vi "Main.vi"() -> ()   [LabVIEW 2018]
doc: "This Continuous Measurement sample project is based on the Queued Message Handler template.\n\nThe Event Handling Loop generates messages based on user interface actions.\n\nThe Message Handling Loop processes messages generated by the Event Handling Loop, or by other messages. There are also Acquisition and Logging message handling loop subVIs, and a chart updating loop."
uses:
  Controls/Acquired Data.ctl
  Settings/Settings.ctl
  Acquisition/Hardware Configuration.ctl
  Acquisition/Signal Type.ctl
  Logging/Logging Configuration.ctl
  Controls/UI State.ctl
  Support/Message Queue/Enqueue Message (Single).vi
  Support/Message Queue/Enqueue Message (Array).vi
  <vilib>/Utility/error.llb/Error Cluster From Error Code.vi
  <vilib>/ErrorRing/Error Ring.xnode
  Acquisition/Acquisition.lvlib
  Logging/Logging.lvlib
  Settings/Settings.lvlib
  support/User Event - Stop/User Event - Stop.lvlib
  support/Message Queue/Message Queue.lvlib
  Settings/Settings Dialog.vi
  Data Display/Data Display.lvlib
panel:
  in  "Data":T1
  out "User Event - Stop":refnum<user-event>
  out "Data":T1(graph)
  in  "Settings":bool
  in  "Start":bool
  in  "Stop":bool
  out "Status":string
  in  "Exit":bool
  # "Continuous Measurement Data Logger"
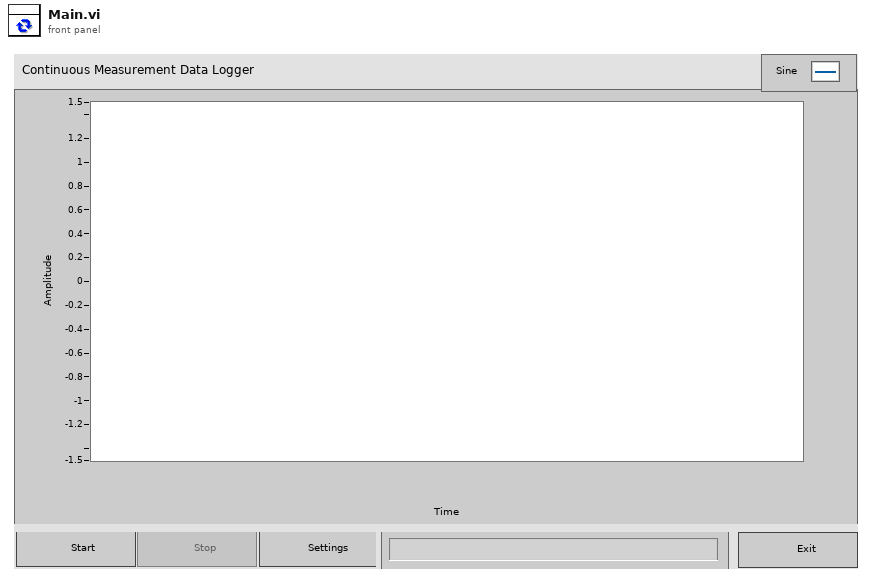
[diagram p1: front panel]
types:
  T1 = typedef "Acquired Data.ctl" = waveform(dbl)[]
  T2 = typedef "UI State.ctl" = enum16{"Idle", "Acquiring and Logging", "Waiting for Exit", "Waiting for Exit (Acq Stopped)", "Waiting for Exit (Log Stopped)", "Waiting for Stop", "Waiting for Stop (Acq Stopped)", "Waiting for Stop (Log Stopped)"}
  T3 = typedef "Settings.lvlib/Settings.ctl" = cluster{"Hardware Configuration":T4, "Logging Configuration":T6, "UI Refs":cluster{"Start Ref":refnum<vi>, "Settings Ref":refnum<vi>, "Stop Ref":refnum<vi>, "Exit Ref":refnum<vi>, "Status Ref":refnum<vi>, "Data Ref":refnum<vi>}}
  T4 = typedef "Acquisition.lvlib/Hardware Configuration.ctl" = cluster{"HW Refnum <Replace Me>":string, "Signal Type <Replace Me>":T5}
  T5 = typedef "Acquisition.lvlib/Signal Type.ctl" = enum16{"Sine Wave", "Square with Noise"}
  T6 = typedef "Logging.lvlib/Logging Configuration.ctl" = cluster{"Log File Base Path":path, "TDMS File Reference":refnum<k34>}
  T7 = typedef "Message Queue.lvlib/All Message Queues.ctl" = cluster{"Message Queues":cluster{"UI":refnum<queue>, "Acquisition":refnum<queue>, "Logging":refnum<queue>}, "Data Queues & Notifier":cluster{"Data Queue":T8, "Data Notifer":T9}}
  T8 = typedef "Data Queue.ctl" = refnum<queue>
  T9 = typedef "Data Notifier.ctl" = refnum<notifier>
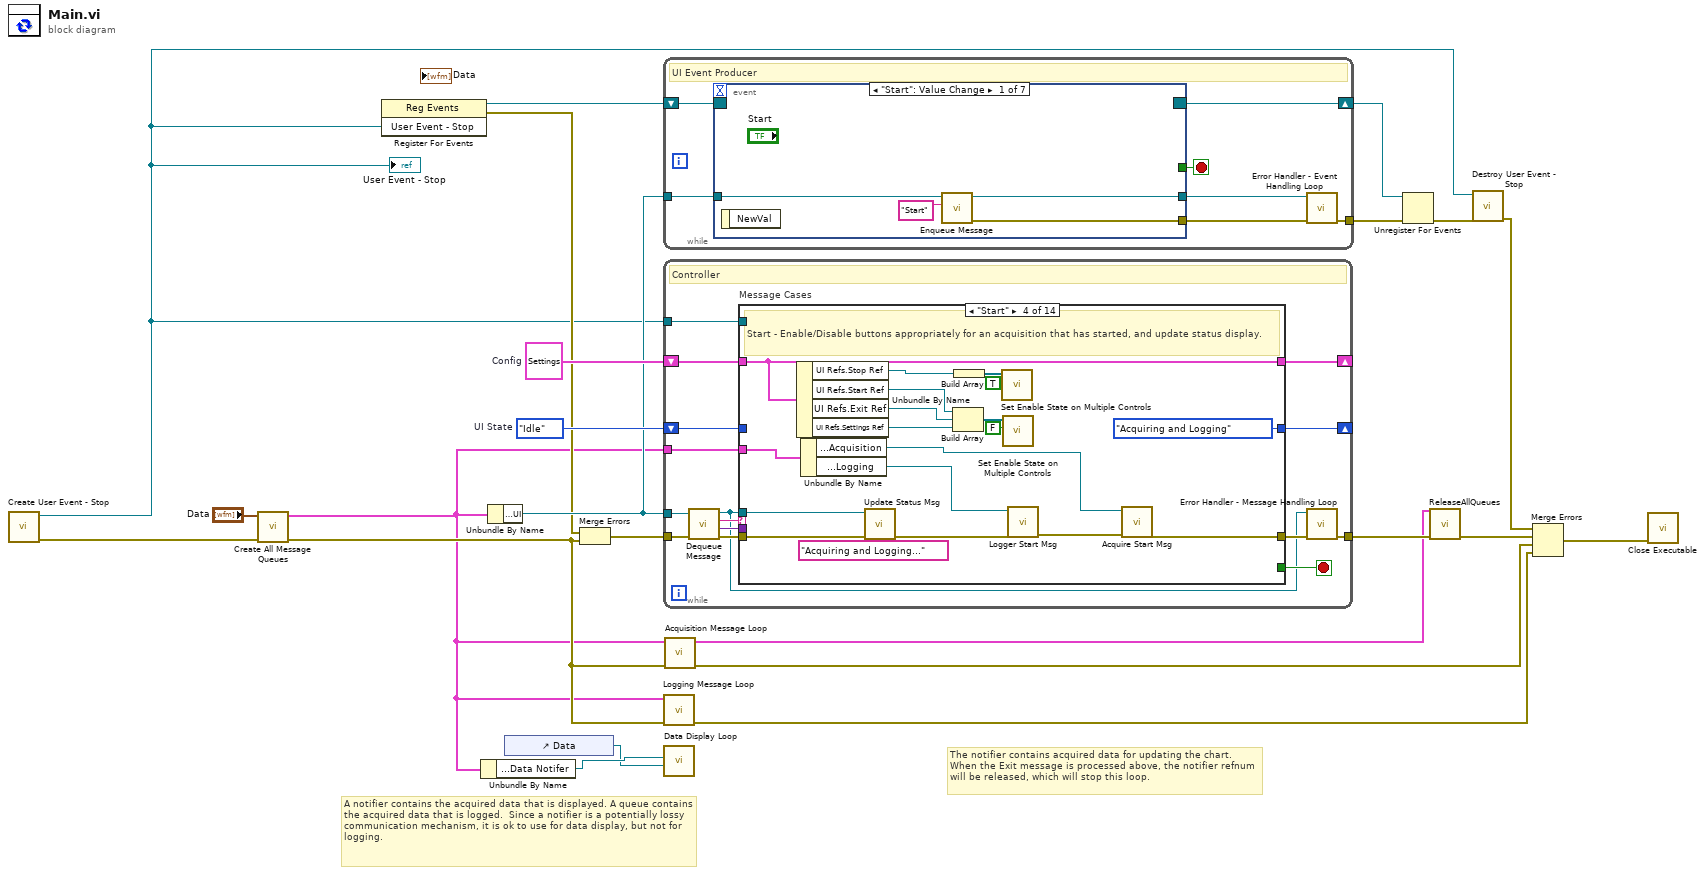
[diagram p0: block diagram]
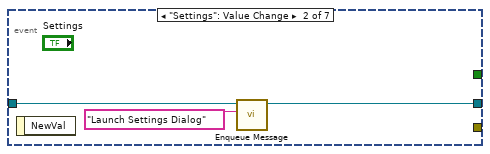
[diagram p2: hidden frame]
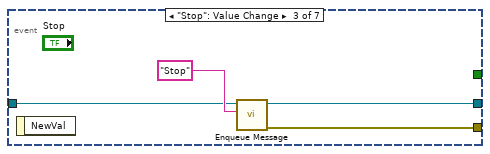
[diagram p3: hidden frame]
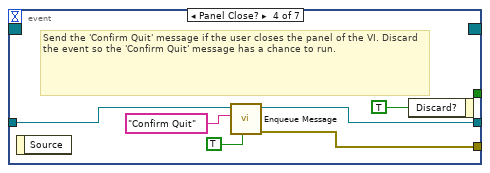
[diagram p4: hidden frame]
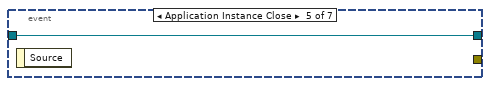
[diagram p5: hidden frame]
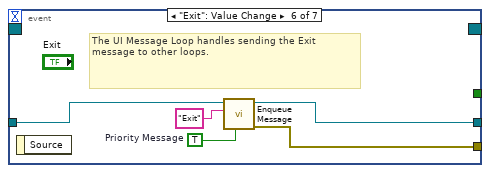
[diagram p6: hidden frame]
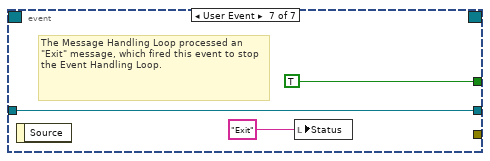
[diagram p7: hidden frame]
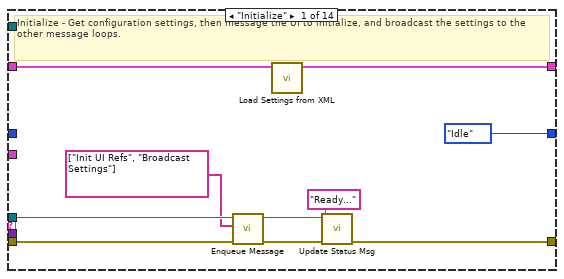
[diagram p8: hidden frame]
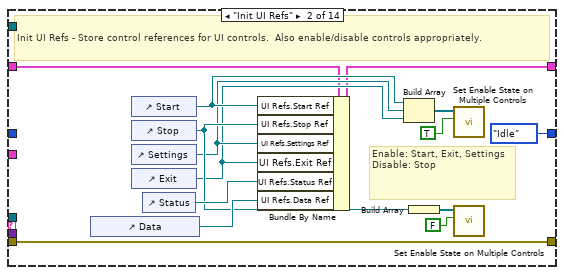
[diagram p9: hidden frame]
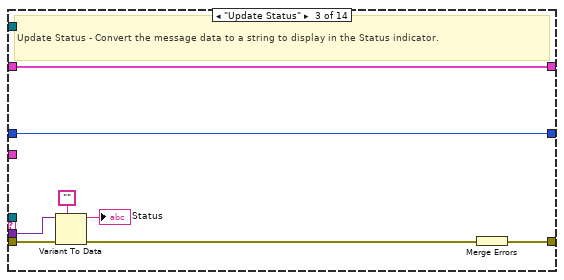
[diagram p10: hidden frame]
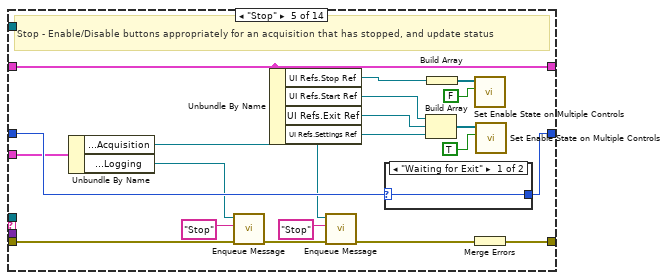
[diagram p11: hidden frame]
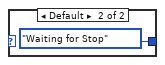
[diagram p12: hidden frame]
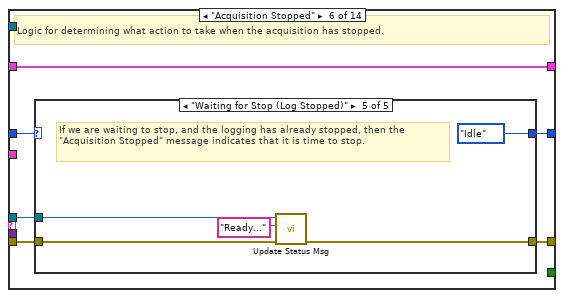
[diagram p13: hidden frame]
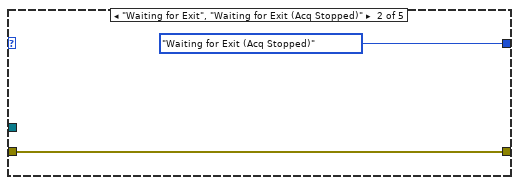
[diagram p15: hidden frame]
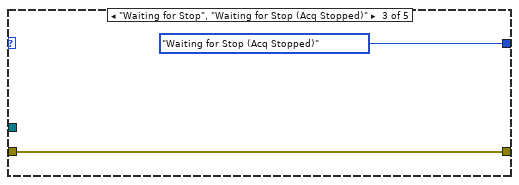
[diagram p16: hidden frame]
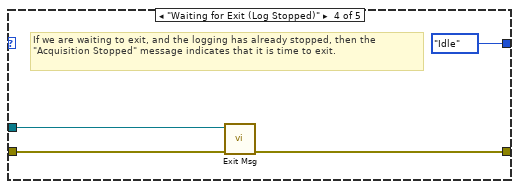
[diagram p17: hidden frame]
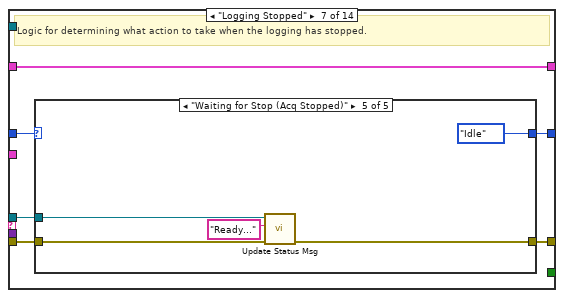
[diagram p18: hidden frame]
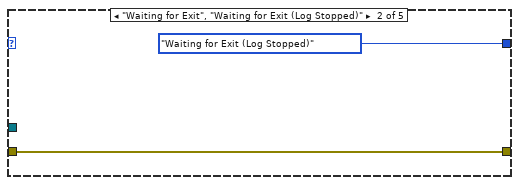
[diagram p20: hidden frame]
diagram:
  w14 = UI_State."Idle"  # UI State
  w16 = T3 {"Hardware Configuration"={"HW Refnum <Replace Me>"="", "Signal Type <Replace Me>"=enum."Sine Wave"}, "Logging Configuration"={"Log File Base Path"=path "", "TDMS File Reference"=refnum}, "UI Refs"={"Start Ref"=refnum, "Settings Ref"=refnum, "Stop Ref"=refnum, "Exit Ref"=refnum, "Status Ref"=refnum, "Data Ref"=refnum}}  # Config
  # "A notifier contains the acquired data that is displayed. A queue contains the acquired data that is logged.  Since a notifier is a potentially lossy communication mechanism, it is ok to use for data display, but not for logging."
  # "The notifier contains acquired data for updating the chart. When the Exit message is processed above, the notifier refnum will be released, which will stop this loop."
  n1 = call "Create User Event - Stop.vi"() -> ("error out"=w19:errorcluster, "User Event - Stop"=w8:refnum<user-event>)  [unwired: 10 in]
  "User Event - Stop" <- w8
  n2 = call "Create All Message Queues.vi"("error in (no error)"=w19, "Data"="Data") -> ("error out"=w17:errorcluster, "Message Queues out"=w5:T7)  [unwired: 8 in]
  n3 = register-events(w8) -> (reference out=w11:refnum<event-registration>, error out=w9:errorcluster)  [unwired: 2 in]
  n4 = Unbundle By Name(w5) -> ("Data Queues & Notifier.Data Notifer"=w7:T9)
  n5 = Unbundle By Name(w5) -> ("Message Queues.UI"=w13:refnum<queue>)
  n6 = control-ref of="Data"() -> (w1:refnum<vi>)
  n7 = Merge Errors(w9, w17) -> (w10:errorcluster)
  n8 = while {
    tunnel: w13 -> [w28]
    tunnel: [w25] -> w21
    shift-right: [w27] -> w15
    shift-left: w11 -> [w29]
    stop <- w26 stop-if-true
    # "UI Event Producer"
    n9 = event shown="[0] \"Start\": Value Change" {
      selector: w29 -> [_ _ _ _ _ _ _]
      dyn-events: [_ _ _ _ _ _ _] -> w27
      timeout: _ -> [_ _ _ _ _ _ _]
      tunnel: [_ _ _ _ _ _ TRUE ("Discard?")] -> w26
      tunnel: w28 -> [w33 w35 w39 w44 w47 w49 w53]
      tunnel: [w31 _ w38 w42 _ w52 _] -> w24
      tunnel: [w30 w34 w37 w43 w47 w48 w53] -> w23
      event "Start": Value Change {
        n10 = event-data() -> ()  [unwired: 1 in, 1 out]
        n11 = call-poly "Enqueue Message.vi"("Message"="Start", "Message Queue"=w33) -> ("error out"=w31:errorcluster, "dup Message Queue"=w30:refnum<queue>)  [unwired: 8 in]
      }
      event "Settings": Value Change {
        n12 = event-data() -> ()  [unwired: 1 in, 1 out]
        n13 = call-poly "Enqueue Message.vi"("Message"="Launch Settings Dialog", "Message Queue"=w35) -> ("dup Message Queue"=w34:refnum<queue>)  [unwired: 8 in, 1 out]
      }
      event "Stop": Value Change {
        n14 = event-data() -> ()  [unwired: 1 in, 1 out]
        n15 = call-poly "Enqueue Message.vi"("Message"="Stop", "Message Queue"=w39) -> ("error out"=w38:errorcluster, "dup Message Queue"=w37:refnum<queue>)  [unwired: 8 in]
      }
      event Panel Close? {
        # "Send the 'Confirm Quit' message if the user closes the panel of the VI. Discard the event so the 'Confirm Quit' message has a chance to run."
        n16 = event-data() -> ()  [unwired: 1 in, 1 out]
        n17 = call-poly "Enqueue Message.vi"("Priority Message? (F)"=TRUE, "Message"="Confirm Quit", "Message Queue"=w44) -> ("error out"=w42:errorcluster, "dup Message Queue"=w43:refnum<queue>)  [unwired: 7 in]
        n18 = event-data("Discard?"=TRUE) -> ()  [unwired: 1 in, 1 out]
      }
      event Application Instance Close {
        n19 = event-data() -> ()  [unwired: 1 in, 1 out]
      }
      event "Exit": Value Change {
        w50 = TRUE  # Priority Message
        # "The UI Message Loop handles sending the Exit message to other loops."
        n20 = event-data() -> ()  [unwired: 1 in, 1 out]
        n21 = call-poly "Enqueue Message.vi"("Priority Message? (F)"=w50, "Message"="Exit", "Message Queue"=w49) -> ("error out"=w52:errorcluster, "dup Message Queue"=w48:refnum<queue>)  [unwired: 7 in]
      }
      event User Event {
        # "The Message Handling Loop processed an \"Exit\" message, which fired this event to stop the Event Handling Loop."
        n22 = event-data() -> ()  [unwired: 1 in, 1 out]
        n23 = local write "Status"("Exit" ("Exit String")) -> ()
      }
    }
    n24 = call "Error Handler - Event Handling Loop.vi"("error in (no error)"=w24, "Message Queue"=w23) -> ("dup error in"=w25:errorcluster)  [unwired: 8 in, 1 out]
  }
  n25 = while {
    tunnel: w13 -> [w64]
    tunnel: w8 -> [w69]
    shift-right: [w63] -> _
    shift-left: w16 -> [w62]
    shift-right: [w57] -> _
    shift-left: w14 -> [w58]
    tunnel: w10 -> [w68]
    tunnel: [w61] -> w22
    tunnel: w5 -> [w56]
    stop <- w70 stop-if-true
    # "Controller"
    n26 = call "Dequeue Message.vi"("error in (no error)"=w68, "Message Queue"=w64) -> ("error out"=w67:errorcluster, "Message Data"=w65:variant, "Message"=w66:string, "dup Message Queue"=w59:refnum<queue>)  [unwired: 6 in]
    n27 = case "Message Cases" shown="\"Start\"" w66 {
      selector: w66 -> [_ _ _ _ _ _ _ _ _ _ _ _ _ w266]
      tunnel: w59 -> [w78 _ _ w106 _ w146 w167 _ w202 _ w221 _ _ _]
      tunnel: w67 -> [w77 w94 w101 w105 w140 w147 w168 w191 w204 w210 w220 w251 w264 _]
      tunnel: [w71 w94 w102 w112 w141 w144 w165 w197 w198 w213 w219 w258 w263 w265] -> w60
      tunnel: [_ _ _ _ _ _ _ _ _ _ _ TRUE _ _] -> w70
      tunnel: w65 -> [_ _ w100 _ _ _ _ _ _ w214 _ w249 _ _]
      tunnel: w69 -> [_ _ _ _ _ _ _ _ _ _ _ w259 _ _]
      tunnel: [w79 w81 w96 w110 w125 w149 w170 w195 w201 w217 w223 w257 w262 w268] -> w63
      tunnel: w62 -> [w80 w82 w96 w110 w125 w149 w170 w195 w205 w217 w223 w257 w262 w268]
      tunnel: w58 -> [_ _ w95 _ w126 w148 w169 w189 w199 w212 w222 _ w261 w267]
      tunnel: [UI_State."Idle" ("UI State") UI_State."Idle" ("UI State") w95 UI_State."Acquiring and Logging" ("UI State") w127 w145 w166 w189 w199 w212 w218 UI_State."Idle" ("UI State") w261 w267] -> w57
      tunnel: w56 -> [_ _ _ w109 w124 _ _ w188 _ _ _ w247 _ _]
      frame "Initialize" {
        # "Initialize - Get configuration settings, then message the UI to initialize, and broadcast the settings to the other message loops."
        n28 = call-poly "Enqueue Message.vi"("error in (no error)"=w77, "Message Array"=string[] ["Init UI Refs", "Broadcast Settings"], "Message Queue"=w78) -> ("error out"=w72:errorcluster, "dup Message Queue"=w74:refnum<queue>)  [unwired: 7 in]
        n29 = call "Load Settings from XML.vi"("Settings in"=w80) -> ("Settings out"=w79:T3)  [unwired: 9 in, 1 out]
        n30 = call "Update Status Msg.vi"("error in (no error)"=w72, "Ready..."="Ready...", "Queue in"=w74) -> ("error out"=w71:errorcluster)  [unwired: 8 in]
      }
      frame "Init UI Refs" {
        # "Enable: Start, Exit, Settings\nDisable: Stop"
        # "Init UI Refs - Store control references for UI controls.  Also enable/disable controls appropriately."
        n31 = control-ref of="Data"() -> (w92:refnum<vi>)
        n32 = control-ref of="Start"() -> (w86:refnum<vi>)
        n33 = control-ref of="Stop"() -> (w87:refnum<vi>)
        n34 = control-ref of="Settings"() -> (w85:refnum<vi>)
        n35 = control-ref of="Exit"() -> (w84:refnum<vi>)
        n36 = control-ref of="Status"() -> (w93:refnum<vi>)
        n37 = Bundle By Name(cluster=w82, "UI Refs.Start Ref"=w86, "UI Refs.Stop Ref"=w87, "UI Refs.Settings Ref"=w85, "UI Refs.Exit Ref"=w84, "UI Refs.Status Ref"=w93, "UI Refs.Data Ref"=w92) -> (w81:T3)
        n38 = Build Array(w86, w85, w84) -> (w90:refnum<vi>[])
        n39 = Build Array(w87) -> (w89:refnum<vi>[])
        n40 = call "Set Enable State on Multiple Controls.vi"("Enable?"=TRUE, "Controls"=w90) -> ()  [unwired: 10 in]
        n41 = call "Set Enable State on Multiple Controls.vi"("Enable?"=FALSE, "Controls"=w89) -> ()  [unwired: 10 in]
      }
      frame "Update Status" {
        # "Update Status - Convert the message data to a string to display in the Status indicator."
        n42 = Variant To Data(error in=w101, type="", Variant=w100) -> (data=→"Status":string, error out=w98:errorcluster)
        n43 = Merge Errors(w98) -> (w102:errorcluster)
      }
      frame "Start" {
        # "Start - Enable/Disable buttons appropriately for an acquisition that has started, and update status display."
        n44 = Unbundle By Name(w110) -> ("UI Refs.Stop Ref"=w117:refnum<vi>, "UI Refs.Start Ref"=w116:refnum<vi>, "UI Refs.Exit Ref"=w115:refnum<vi>, "UI Refs.Settings Ref"=w114:refnum<vi>)
        n45 = Unbundle By Name(w109) -> ("Message Queues.Acquisition"=w108:refnum<queue>, "Message Queues.Logging"=w107:refnum<queue>)
        n46 = call "Update Status Msg.vi"("error in (no error)"=w105, "Ready..."="Acquiring and Logging..." ("Acquiring and Logging..."), "Queue in"=w106) -> ("error out"=w104:errorcluster)  [unwired: 8 in]
        n47 = Build Array(w116, w115, w114) -> (w120:refnum<vi>[])
        n48 = Build Array(w117) -> (w119:refnum<vi>[])
        n49 = call "Set Enable State on Multiple Controls.vi"("Enable?"=TRUE, "Controls"=w119) -> ()  [unwired: 10 in]
        n50 = call "Set Enable State on Multiple Controls.vi"("Enable?"=FALSE, "Controls"=w120) -> ()  [unwired: 10 in]
        n51 = call "Logger Start Msg.vi"("error in (no error)"=w104, "Queue in"=w107) -> ("error out"=w113:errorcluster)  [unwired: 9 in]
        n52 = call "Acquire Start Msg.vi"("error in (no error)"=w113, "Queue in"=w108) -> ("error out"=w112:errorcluster)  [unwired: 9 in]
      }
      frame "Stop" {
        # "Stop - Enable/Disable buttons appropriately for an acquisition that has stopped, and update status"
        n53 = Unbundle By Name(w124) -> ("Message Queues.Acquisition"=w123:refnum<queue>, "Message Queues.Logging"=w122:refnum<queue>)
        n54 = call-poly "Enqueue Message.vi"("error in (no error)"=w140, "Message"="Stop", "Message Queue"=w122) -> ("error out"=w130:errorcluster)  [unwired: 7 in, 1 out]
        n55 = Unbundle By Name(w125) -> ("UI Refs.Stop Ref"=w135:refnum<vi>, "UI Refs.Start Ref"=w134:refnum<vi>, "UI Refs.Exit Ref"=w133:refnum<vi>, "UI Refs.Settings Ref"=w132:refnum<vi>)
        n56 = call-poly "Enqueue Message.vi"("error in (no error)"=w130, "Message"="Stop", "Message Queue"=w123) -> ("error out"=w129:errorcluster)  [unwired: 7 in, 1 out]
        n57 = case shown="\"Waiting for Exit\"" w126 {
          selector: w126 -> [w142 _]
          tunnel: [w142 UI_State."Waiting for Stop" ("UI State")] -> w127
          frame "Waiting for Exit" {
          }
          frame Default {
          }
        }
        n58 = Build Array(w134, w133, w132) -> (w138:refnum<vi>[])
        n59 = Build Array(w135) -> (w137:refnum<vi>[])
        n60 = call "Set Enable State on Multiple Controls.vi"("Enable?"=FALSE, "Controls"=w137) -> ()  [unwired: 10 in]
        n61 = Merge Errors(w129) -> (w141:errorcluster)
        n62 = call "Set Enable State on Multiple Controls.vi"("Enable?"=TRUE, "Controls"=w138) -> ()  [unwired: 10 in]
      }
      frame "Acquisition Stopped" {
        # "Logic for determining what action to take when the acquisition has stopped."
        n63 = case shown="\"Waiting for Stop (Log Stopped)\"" w148 {
          selector: w148 -> [w151 _ _ _ _]
          tunnel: w147 -> [w150 w153 w155 w158 w162]
          tunnel: w146 -> [_ _ _ w157 w163]
          tunnel: [w151 UI_State."Waiting for Exit (Acq Stopped)" ("UI State") UI_State."Waiting for Stop (Acq Stopped)" ("UI State") UI_State."Idle" ("UI State") UI_State."Idle" ("UI State")] -> w145
          tunnel: [w150 w153 w155 w156 w161] -> w144
          frame Default {
          }
          frame "Waiting for Exit", "Waiting for Exit (Acq Stopped)" {
          }
          frame "Waiting for Stop", "Waiting for Stop (Acq Stopped)" {
          }
          frame "Waiting for Exit (Log Stopped)" {
            # "If we are waiting to exit, and the logging has already stopped, then the \"Acquisition Stopped\" message indicates that it is time to exit."
            n64 = call "Exit Msg.vi"("error in (no error)"=w158, "Queue in"=w157) -> ("error out"=w156:errorcluster)  [unwired: 9 in]
          }
          frame "Waiting for Stop (Log Stopped)" {
            # "If we are waiting to stop, and the logging has already stopped, then the \"Acquisition Stopped\" message indicates that it is time to stop."
            n65 = call "Update Status Msg.vi"("error in (no error)"=w162, "Ready..."="Ready...", "Queue in"=w163) -> ("error out"=w161:errorcluster)  [unwired: 8 in]
          }
        }
      }
      frame "Logging Stopped" {
        # "Logic for determining what action to take when the logging has stopped."
        n66 = case shown="\"Waiting for Stop (Acq Stopped)\"" w169 {
          selector: w169 -> [w172 _ _ _ _]
          tunnel: w168 -> [w171 w174 w176 w180 w183]
          tunnel: w167 -> [_ _ _ w178 w182]
          tunnel: [w172 UI_State."Waiting for Exit (Log Stopped)" ("UI State") UI_State."Waiting for Stop (Log Stopped)" ("UI State") UI_State."Idle" ("UI State") UI_State."Idle" ("UI State")] -> w166
          tunnel: [w171 w174 w176 w179 w181] -> w165
          frame Default {
          }
          frame "Waiting for Exit", "Waiting for Exit (Log Stopped)" {
          }
          frame "Waiting for Stop", "Waiting for Stop (Log Stopped)" {
          }
          frame "Waiting for Exit (Acq Stopped)" {
            n67 = call "Exit Msg.vi"("error in (no error)"=w180, "Queue in"=w178) -> ("error out"=w179:errorcluster)  [unwired: 9 in]
          }
          frame "Waiting for Stop (Acq Stopped)" {
            n68 = call "Update Status Msg.vi"("error in (no error)"=w183, "Ready..."="Ready...", "Queue in"=w182) -> ("error out"=w181:errorcluster)  [unwired: 8 in]
          }
        }
      }
      frame "Broadcast settings" {
        w190 = "Update Settings" ("Message")
        # "Broadcast settings - Send the 'Update Settings' message to the Logging and Acquisition message loops."
        n69 = Unbundle By Name(w195) -> ("Hardware Configuration"=w194:T4, "Logging Configuration"=w193:T6)
        n70 = Unbundle By Name(w188) -> ("Message Queues.Acquisition"=w187:refnum<queue>, "Message Queues.Logging"=w186:refnum<queue>)
        n71 = call-poly "Enqueue Message.vi"("Message Data"=w194, "Message"=w190, "Message Queue"=w187) -> ("error out"=w196:errorcluster)  [unwired: 7 in, 1 out]
        n72 = call-poly "Enqueue Message.vi"("error in (no error)"=w196, "Message Data"=w193, "Message"=w190, "Message Queue"=w186) -> ("error out"=w192:errorcluster)  [unwired: 6 in, 1 out]
        n73 = Merge Errors(w192, w191) -> (w197:errorcluster)
      }
      frame "Launch Settings Dialog" {
        # "Launch Settings Dialog - Launch the Settings Dialog when the user clicks the 'Settings' button."
        n74 = call-by-ref "?"("error in (no error)"=w204, "Settings in"=w205) -> ("error out"=w200:errorcluster, "Cancelled?"=w203:bool, "Settings out"=w201:T3)  [unwired: 8 in, 3 out]
        n75 = case shown="False" w203 {
          tunnel: w202 -> [w208 _]
          tunnel: w200 -> [w207 w209]
          tunnel: [w206 w209] -> w198
          frame False {
            n76 = call "Broadcast Settings Msg.vi"("error in (no error)"=w207, "Queue in"=w208) -> ("error out"=w206:errorcluster)  [unwired: 9 in]
          }
          frame True {
          }
        }
      }
      frame "Error" {
        # "Error - Display an error dialog. This message is sent by the \"Error Handler\" VIs at the end of other loops in this application."
        n77 = Variant To Data(error in=w210, type=errorcluster {"status"=FALSE, "code"=0, "source"=""} ("error constant"), Variant=w214) -> (data=w211:errorcluster, error out=w215:errorcluster)
        n78 = call <vilib>:"Simple Error Handler.vi"("error in (no error)"=w211) -> ()  [unwired: 4 in, 5 out]
        n79 = Merge Errors(w215) -> (w213:errorcluster)
      }
      frame "Confirm Quit" {
        # "Confirm Quit - Message that can confirm whether or not the user wants to exit the application."
        n80 = case shown="\"Acquiring and Logging\"" w222 {
          tunnel: w221 -> [w229 w233]
          tunnel: w220 -> [w228 w232]
          tunnel: [w227 w231] -> w219
          tunnel: [UI_State."Idle" ("UI State") w230] -> w218
          frame Default {
            # "If 'Confirm Quit' comes in while the system is idle, there is no need for a confirmation message."
            n81 = call-poly "Enqueue Message.vi"("Priority Message? (F)"=TRUE, "error in (no error)"=w228, "Message"="Exit", "Message Queue"=w229) -> ("error out"=w227:errorcluster)  [unwired: 6 in, 1 out]
          }
          frame "Acquiring and Logging" {
            n82 = Two Button Dialog(message="Are you sure you want to quit while the acquisition is running?" ("Confirm Quit Message"), 1:"No" ("No"), 2:"Yes" ("Yes")) -> (T button?=w234:bool)
            n83 = case shown="True" w234 {
              tunnel: w233 -> [_ w242]
              tunnel: w232 -> [w239 w243]
              tunnel: [w239 w241] -> w231
              tunnel: [UI_State."Acquiring and Logging" ("UI State") UI_State."Waiting for Exit" ("UI State")] -> w230
              frame False {
                # "User did not want to quit."
              }
              frame True {
                n84 = call "Stop Msg.vi"("error in (no error)"=w243, "Queue in"=w242) -> ("error out"=w241:errorcluster)  [unwired: 9 in]
              }
            }
          }
        }
      }
      frame "Exit" {
        w254 = "Exit" ("Message")
        # "Popup an error dialog if 'Exit' was called as a result of an error."
        # "Stop the VI"
        # "Exit - Send Exit messages to the Acquisition and Logging loops, and fire the user event to stop the Event Handling Loop."
        n85 = Unbundle By Name(w247) -> ("Message Queues.Acquisition"=w246:refnum<queue>, "Message Queues.Logging"=w245:refnum<queue>)
        n86 = Variant To Data(type=errorcluster {"status"=FALSE, "code"=0, "source"=""} ("error constant"), Variant=w249) -> (data=w248:errorcluster)  [unwired: 1 in, 1 out]
        n87 = call <vilib>:"Simple Error Handler.vi"("error in (no error)"=w248) -> ()  [unwired: 4 in, 5 out]
        n88 = call-poly "Enqueue Message.vi"("Priority Message? (F)"=TRUE, "error in (no error)"=w251, "Message"=w254, "Message Queue"=w246) -> ("error out"=w255:errorcluster)  [unwired: 6 in, 1 out]
        n89 = call-poly "Enqueue Message.vi"("Priority Message? (F)"=TRUE, "error in (no error)"=w255, "Message"=w254, "Message Queue"=w245) -> ("error out"=w252:errorcluster)  [unwired: 6 in, 1 out]
        n90 = call "Fire User Event - Stop.vi"("error in (no error)"=w252, "User Event - Stop"=w259) -> ("error out"=w258:errorcluster)  [unwired: 9 in]
      }
      frame "---Copy This Frame---" {
        # "Duplicate this frame when creating new messages.  Change this comment in the duplicated frame to describe this message."
        n91 = Merge Errors(w264) -> (w263:errorcluster)
      }
      frame Default {
        # "'Default' case only runs if there is a message that isn't defined in any of the other cases.  Output a programming error."
        n92 = xnode "Error Ring"("parameter 0"=w266) -> ("error out"=w265:errorcluster)
      }
    }
    n93 = call "Error Handler - Message Handling Loop.vi"("error in (no error)"=w60, "Message Queue"=w59) -> ("dup error in"=w61:errorcluster)  [unwired: 8 in, 1 out]
  }
  n94 = call "Logging Message Loop.vi"("error in (no error)"=w17, "Message Queues"=w5) -> ("error out"=w18:errorcluster)  [unwired: 9 in]
  n95 = call "Data Display Loop.vi"("Data"=w1, "Notifier in"=w7) -> ()  [unwired: 10 in]
  n96 = call "Acquisition Message Loop.vi"("error in (no error)"=w17, "Message Queues"=w5) -> ("error out"=w20:errorcluster)  [unwired: 9 in]
  n97 = Unregister For Events(event registration refnum=w15, error in=w21) -> (error out=w3:errorcluster)
  n98 = call "ReleaseAllQueues.vi"("error in (no error)"=w22, "Message Queues"=w5) -> ("error out"=w12:errorcluster)  [unwired: 9 in]
  n99 = call "Destroy User Event - Stop.vi"("error in (no error)"=w3, "User Event - Stop"=w8) -> ("error out"=w2:errorcluster)  [unwired: 9 in]
  n100 = Merge Errors(w2, w12, w20, w18) -> (w4:errorcluster)
  n101 = call "Close Executable.vi"("error in (no error)"=w4) -> ()  [unwired: 11 in]
